vi "Check for Serial Input Channel Error.vi"(0 "serial input channel status":T1[](array[typedef])=[{"acq state"=enum."Idle", "stop timed out"=FALSE, "bad packet header"=FALSE, "bad packet payload"=FALSE, "bad packet size"=FALSE, "dram status"={"bytes written"=0, "bytes read"=0, "overflow"=FALSE, "partition full"=FALSE, "last byte flushed"=FALSE}}, {"acq state"=enum."Idle", "stop timed out"=FALSE, "bad packet header"=FALSE, "bad packet payload"=FALSE, "bad packet size"=FALSE, "dram status"={"bytes written"=0, "bytes read"=0, "overflow"=FALSE, "partition full"=FALSE, "last byte flushed"=FALSE}}, {"acq state"=enum."Idle", "stop timed out"=FALSE, "bad packet header"=FALSE, "bad packet payload"=FALSE, "bad packet size"=FALSE, "dram status"={"bytes written"=0, "bytes read"=0, "overflow"=FALSE, "partition full"=FALSE, "last byte flushed"=FALSE}}, {"acq state"=enum."Idle", "stop timed out"=FALSE, "bad packet header"=FALSE, "bad packet payload"=FALSE, "bad packet size"=FALSE, "dram status"={"bytes written"=0, "bytes read"=0, "overflow"=FALSE, "partition full"=FALSE, "last byte flushed"=FALSE}}]) -> (4 "acquisition error":bool)   [LabVIEW 2020, in "GettingStarted_Acq_Tap_148X_FPGA.lvlib"]
uses:
  GettingStarted_Acq_Tap_148X_FPGA.lvlib
  Types/Serial Input Channel Status.ctl
  <instrlib>/FlexRIO/CSI-2/v2/FPGA/Types/Channel-Based Acquisition Engine State.ctl
  Common/Types/DRAM Status.ctl
  <instrlib>/FlexRIO/CSI-2/v2/FPGA/NI CSI-2 API FPGA v2.lvlib
  Common/GettingStarted_Common_148X_FPGA.lvlib
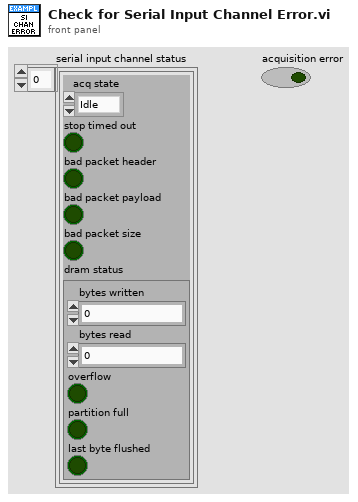
[diagram p1: front panel]
types:
  T1 = typedef "GettingStarted_Acq_Tap_148X_FPGA.lvlib/Serial Input Channel Status.ctl" = cluster{"acq state":T2, "stop timed out":bool, "bad packet header":bool, "bad packet payload":bool, "bad packet size":bool, "dram status":T3}
  T2 = typedef "NI CSI-2 API FPGA v2.lvlib/Channel-Based Acquisition Engine State.ctl" = enum8{"Idle", "Wait for First Packet Header", "Acquire", "Wait for Last Packet Header", "Wait for End of Last Packet"}
  T3 = typedef "GettingStarted_Common_148X_FPGA.lvlib/DRAM Status.ctl" = cluster{"bytes written":u64, "bytes read":u64, "overflow":bool, "partition full":bool, "last byte flushed":bool}
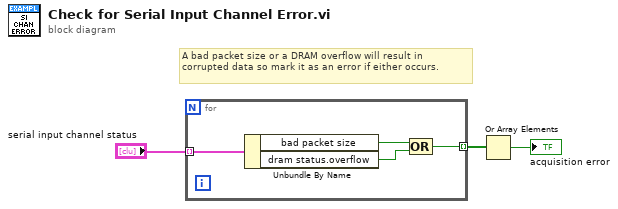
[diagram p0: block diagram]
diagram:
  # "A bad packet size or a DRAM overflow will result in corrupted data so mark it as an error if either occurs."
  n1 = for {
    tunnel: "serial input channel status" -> [w7] mode=indexing
    tunnel: [w4] -> w2 mode=indexing
    n2 = Unbundle By Name(w7) -> ("bad packet size"=w5:bool, "dram status.overflow"=w6:bool)
    n3 = Compound Arithmetic op=OR(w5, w6) -> (w4:bool)
  }
  n4 = Or Array Elements(Boolean array=w2) -> (logical OR=→"acquisition error":bool)
